vi "主程序.vi"() -> ()   [LabVIEW 2010]
panel:
  out "x(i-3)":dbl
  out "x(i-2)":dbl
  out "x(i-1)":dbl
  out "x(i)":dbl
  in  "?":bool
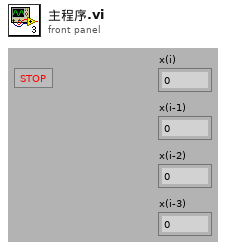
[diagram p1: front panel]
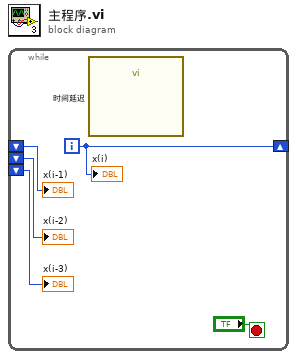
[diagram p0: block diagram]
diagram:
  n1 = while {
    shift-right: [w4] -> _
    shift-left: _ -> [w3]
    shift-left: _ -> [w2]
    shift-left: _ -> [w1]
    i -> [w4]
    stop <- "?" stop-if-true
    n2 = call "时间延迟"() -> ()  [unwired: 11 in, 1 out]
    "x(i)" <- w4
    "x(i-1)" <- w3
    "x(i-2)" <- w2
    "x(i-3)" <- w1
  }
